vi "splash.vi"() -> ()   [LabVIEW 2010]
uses:
  <vilib>/Utility/miscctls.llb/LVRectTypeDef.ctl
  lib/Global 2.vi
  <vilib>/Platform/browser.llb/Open URL in Default Browser (string).vi
panel:
  out "msgs":cluster{"time stamp":timestamp, "t0":string}[](array[cluster]) {"time stamp" format="%<%.1X>T"}
  out "Bool3":bool
  out "Bool2":bool
  out "size(s)":i32 caption="шт"
  out "names":string[](array[string]) caption="Неотправленные"
  in  "Tab Control":T1(tab)
  out "Waveform Graph":waveform(i16)[](graph) caption="Последний кадр"
  out "Waveform Graph 2":waveform(i16)[](graph) caption="Последний кадр"
  out "XY Graph":cluster{dbl[], dbl[]}(graph) caption="неотправлено файлов"
  out "XY2":cluster{dbl[], dbl[]}(graph) caption="использование буфера"
  in  "indexhtm":bool
  out "Array":timestamp[](array[timestamp]) caption="Время событий" format="%<%.7X>T"
  out "Bool":bool
  in  "stop":bool
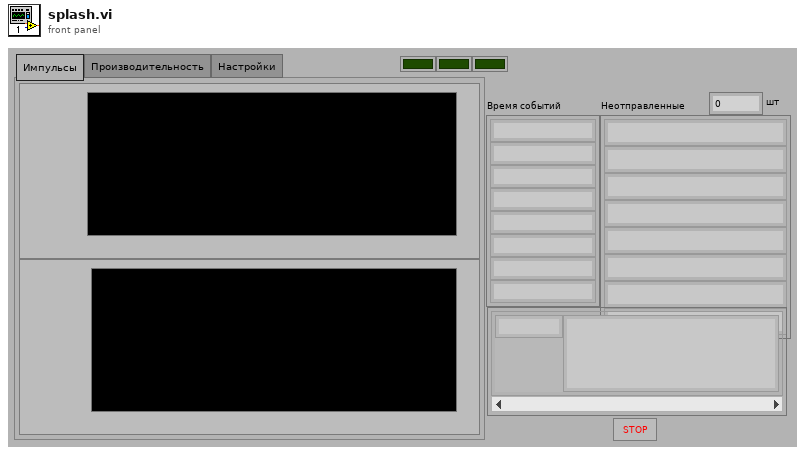
[diagram p1: front panel]
types:
  T1 = enum32{"Импульсы", "Производительность", "Настройки"}
  T2 = enum8{"Enabled", "Disabled", "Disabled and Grayed Out"}
  T3 = typedef "LVRectTypeDef.ctl" = cluster{"Left":i16, "Top":i16, "Right":i16, "Bottom":i16}
  T4 = cluster{"name":enum16{"sync", "phase_a", "phase_b", "phase_c", "ground"}, "num":i32}[]
  T5 = cluster{"seconds since 1Jan1904":timestamp, string}
  T6 = cluster{"seconds since 1Jan1904":timestamp, string}[]
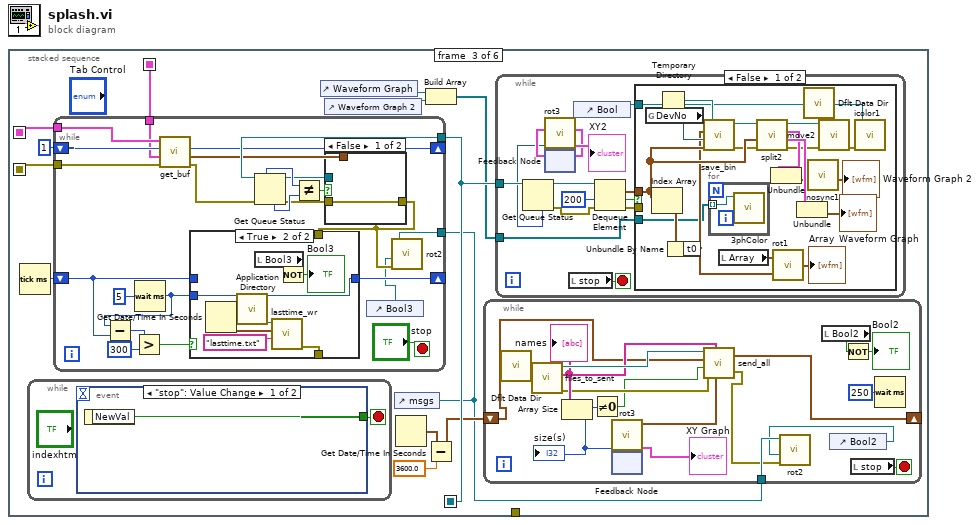
[diagram p0: block diagram]
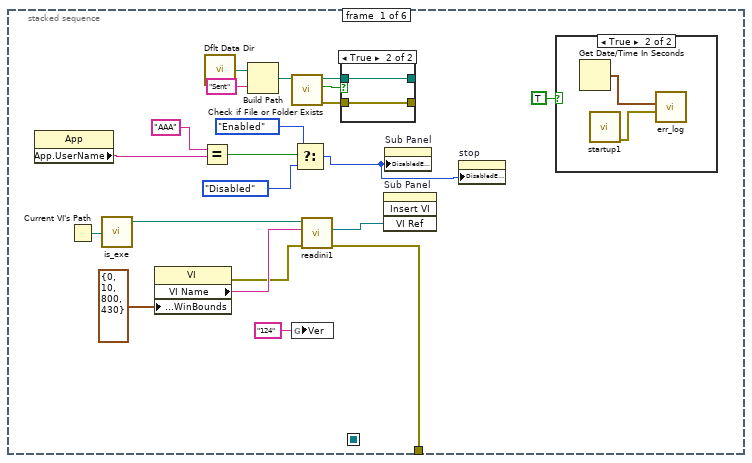
[diagram p2: hidden frame]
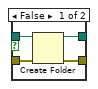
[diagram p4: hidden frame]
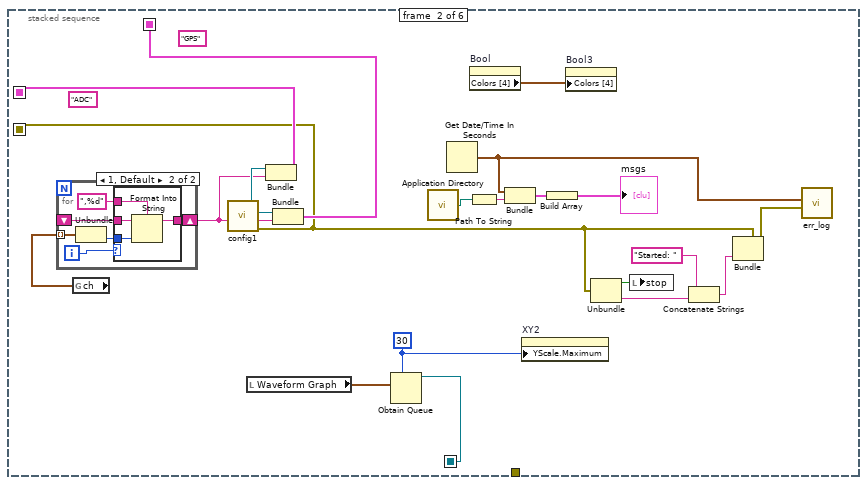
[diagram p5: hidden frame]
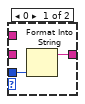
[diagram p6: hidden frame]
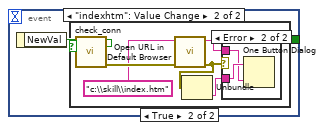
[diagram p7: hidden frame]
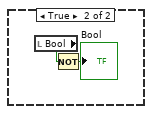
[diagram p10: hidden frame]
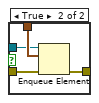
[diagram p12: hidden frame]
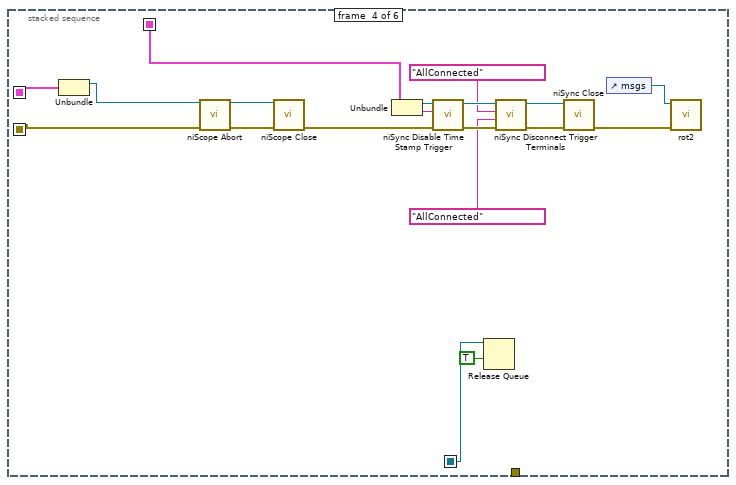
[diagram p13: hidden frame]
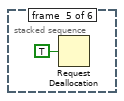
[diagram p14: hidden frame]
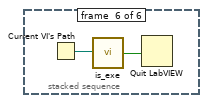
[diagram p15: hidden frame]
diagram:
  n1 = stacked-sequence {
    seq-local: [_ w35 _ _ _ _] -> [_ _ w76 w190 _ _]
    seq-local: [_ w51 _ _ _ _] -> [_ _ w75 w196 _ _]
    seq-local: [_ w45 _ _ _ _] -> [_ _ w73 w184 _ _]
    seq-local: [_ w46 _ _ _ _] -> [_ _ w72 w186 _ _]
    tunnel: [w18 _ _ _ _ _] -> _
    frame #0 {
      n2 = property class="App"() -> ("App.UserName"=w4:string)  [unwired: 2 in, 2 out]
      n3 = Current VI's Path() -> (path=w21:path)
      n4 = call "is_exe.vi"("path"=w21) -> ("ini path"=w19:path)  [unwired: 2 in, 2 out]
      n5 = property class="VI"("Front Panel.WinBounds"=T3 {"Left"=0, "Top"=10, "Right"=800, "Bottom"=430} ("Front Panel Window:Window Bounds")) -> (error out=w17:errorcluster, "VI Name"=w20:string)  [unwired: 2 in, 1 out]
      n6 = Equal?(x="ААА", y=w4) -> (x = y?=w7:bool)
      n7 = call <vilib>:"Dflt Data Dir.vi"() -> ("App:Default Data Directory"=w14:path)
      n8 = Build Path(base path=w14, name or relative path="Sent") -> (appended path=w12:path)
      n9 = call <vilib>:"Check if File or Folder Exists.vi"("path"=w12) -> ("error out"=w9:errorcluster, "file or folder exists?"=w11:bool, "dup path"=w10:path)  [unwired: 8 in]
      n10 = global write "Global 2.vi" "Ver"("124" ("Ver")) -> ()
      n11 = Select(t=T2."Enabled" ("Disabled"), s=w7, f=T2."Disabled" ("Disabled")) -> (s? t:f=w3:T2)
      n12 = call "readini1.vi"("error in (no error)"=w17, "section"=w20, "configuration file path"=w19) -> ("error out"=w18:errorcluster, "ini_reference out"=w15:refnum<vi>)  [unwired: 2 in, 1 out]
      n13 = case shown="True" w11 {
        tunnel: w10 -> [w27 w29]
        tunnel: w9 -> [w26 w28]
        tunnel: [w25 w29] -> _
        tunnel: [w24 w28] -> _
        frame False {
          n14 = Create Folder(path (use dialog)=w27, error in=w26) -> (created path=w25:path, error out=w24:errorcluster)  [unwired: 1 in, 1 out]
        }
        frame True {
        }
      }
      n15 = invoke on="Sub Panel" class="SubPanel" method="Insert VI"("VI Ref"=w15) -> ()  [unwired: 3 in, 4 out]
      n16 = property on="Sub Panel" class="SubPnl"("DisabledEnum"=w3) -> ()  [unwired: 2 in, 2 out]
      n17 = property on="stop" class="Bool (strict)"("DisabledEnum"=w3) -> ()  [unwired: 2 in, 2 out]
      n18 = case shown="True" TRUE {
        frame False {
        }
        frame True {
          n19 = Get Date/Time In Seconds() -> (seconds since 1Jan1904=w22:timestamp)
          n20 = call "startup1.vi"() -> ("error out"=w23:errorcluster)  [unwired: 7 in]
          n21 = call "err_log.vi"("error IO 2"=w23, "time stamp"=w22) -> ()  [unwired: 6 in]
        }
      }
    }
    frame #1 {
      (unwired) "GPS"
      w42 = 30 ("max queue size (-1, unlimited)")
      (unwired) "ADC"
      n22 = global read "Global 2.vi" "ch"() -> (w50:T4)
      n23 = for {
        shift-right: [w55] -> w43
        shift-left: _ -> [w54]
        tunnel: w50 -> [w57] mode=indexing
        i -> [w53]
        n24 = Unbundle(w57) -> ("num"=w56:i32)  [unwired: 1 out]
        n25 = case shown="1, Default" w53 {
          tunnel: w56 -> [w59 w63]
          tunnel: [w58 w62] -> w55
          tunnel: w54 -> [_ w61]
          tunnel: ",%d" -> [_ w60]
          frame 0 {
            n26 = Format Into String(w59) -> (resulting string=w58:string)  [unwired: 3 in, 1 out]
          }
          frame 1, Default {
            n27 = Format Into String(format string=w60, initial string=w61, w63) -> (resulting string=w62:string)  [unwired: 1 in, 1 out]
          }
        }
      }
      n28 = call "config1.vi"("ChList"=w43) -> ("error out"=w35:errorcluster, "trig"=w47:tag, "gps handle"=w48:refnum<k15>, "adc handle"=w49:refnum<k15>)  [unwired: 3 in]
      n29 = local read "Waveform Graph"() -> (w44:waveform(i16)[])
      n30 = Bundle("adc handle"=w49, w43) -> (w46:cluster{"adc handle":refnum<k15>, string})  [unwired: 1 in]
      n31 = Bundle("gps handle"=w48, "trig"=w47) -> (w45:cluster{"gps handle":refnum<k15>, "trig":tag})  [unwired: 1 in]
      n32 = Obtain Queue(max queue size (-1, unlimited)=w42, element data type=w44) -> (queue out=w51:refnum<queue>)  [unwired: 3 in, 2 out]
      n33 = call <vilib>:"Application Directory.vi"() -> ("Application Directory"=w39:path)
      n34 = Get Date/Time In Seconds() -> (seconds since 1Jan1904=w36:timestamp)
      n35 = Path To String(path=w39) -> (string=w41:string)
      n36 = property on="Bool" class="Bool (strict)"() -> ("Colors [4]"=w30:cluster{u32, u32}[])  [unwired: 2 in, 2 out]
      n37 = Bundle("seconds since 1Jan1904"=w36, w41) -> (w40:T5)  [unwired: 1 in]
      n38 = property on="XY2" class="XYGraph (strict)"("YScale.Maximum"=w42) -> ()  [unwired: 2 in, 2 out]
      n39 = Build Array(w40) -> (→"msgs":T6)
      n40 = property on="Bool3" class="Bool (strict)"("Colors [4]"=w30) -> ()  [unwired: 2 in, 2 out]
      n41 = Unbundle(w35) -> ("status"=w38:bool, "source"=w32:string)  [unwired: 1 out]
      n42 = local write "stop"(w38) -> ()
      n43 = Concatenate Strings("Started: " ("string"), w32) -> (w33:string)
      n44 = Bundle(cluster=w35, "source"=w33) -> (w34:errorcluster)  [unwired: 2 in]
      n45 = call "err_log.vi"("error IO 2"=w34, "time stamp"=w36) -> ()  [unwired: 6 in]
    }
    frame #2 {
      n46 = Tick Count (ms)() -> (millisecond timer value=w71:u32)
      n47 = while {
        stop <- w77 stop-if-true
        n48 = event shown="[0] \"stop\": Value Change" {
          selector: _ -> [_ _]
          dyn-events: _ -> [_ _]
          timeout: _ -> [_ _]
          tunnel: [w78 _] -> w77
          event "stop": Value Change {
            n49 = event-data() -> ("NewVal"=w78:bool)  [unwired: 1 in]
          }
          event "indexhtm": Value Change {
            n50 = event-data() -> ("NewVal"=w79:bool)  [unwired: 1 in]
            n51 = case shown="True" w79 {
              frame False {
              }
              frame True {
                n52 = call "check_conn.vi"() -> ("error out"=w81:errorcluster)  [unwired: 6 in, 1 out]
                n53 = call-poly <vilib>:"Open URL in Default Browser.vi"("error in (no error)"=w81, "URL"="c:\\skill\\index.htm") -> ("error out"=w84:errorcluster, "URL out"=w82:string)  [unwired: 4 in]
                n54 = Unbundle(w84) -> ("source"=w83:string)  [unwired: 2 out]
                n55 = case shown="Error" w84 {
                  tunnel: w83 -> [_ w86]
                  tunnel: w82 -> [_ w85]
                  frame No Error {
                  }
                  frame Error {
                    n56 = One Button Dialog(message=w86, button name ("OK")=w85) -> ()  [unwired: 1 out]
                  }
                }
              }
            }
          }
        }
      }
      n57 = control-ref of="Waveform Graph"() -> (w65:refnum<vi>)
      n58 = control-ref of="Waveform Graph 2"() -> (w66:refnum<vi>)
      n59 = control-ref of="msgs"() -> (w67:refnum<vi>)
      n60 = while {
        tunnel: w75 -> [w165]
        tunnel: w76 -> [w154]
        shift-right: [w158] -> _
        shift-left: 1 ("acquisition status out") -> [w157]
        tunnel: w73 -> [w145]
        tunnel: w72 -> [w146]
        shift-right: [w150] -> _
        shift-left: w71 -> [w149]
        tunnel: w67 -> [w144]
        stop <- "stop" stop-if-true
        n61 = Wait (ms)(milliseconds to wait=u32 5) -> (millisecond timer value=w148:u32)
        n62 = Subtract(x=w148, y=w149) -> (x-y=w153:u32)
        n63 = Greater?(x=w153, y=u32 300) -> (0:w152:bool)
        n64 = call "get_buf.vi"("error in"=w154, "Sync cluster"=w145, "acquisition status"=w157, "Scope Cluster"=w146) -> ("error out"=w155:errorcluster, "wfm"=w156:waveform(i16)[], "acquisition status out"=w158:i32)  [unwired: 1 in]
        n65 = Get Queue Status(queue=w165, error in (no error)=w155) -> (queue out=w161:refnum<queue>, max queue size=w164:i32, error out=w160:errorcluster, # elements in queue=w163:i32)  [unwired: 1 in, 4 out]
        n66 = Not Equal?(x=w164, y=w163) -> (x != y?=w162:bool)
        n67 = case shown="False" w162 {
          tunnel: w156 -> [_ w179]
          tunnel: w161 -> [_ w178]
          tunnel: w160 -> [w175 w177]
          tunnel: [w175 w176] -> w143
          frame False {
          }
          frame True {
            n68 = Enqueue Element(queue=w178, element=w179, error in (no error)=w177) -> (error out=w176:errorcluster)  [unwired: 1 in, 2 out]
          }
        }
        n69 = case shown="True" w152 {
          tunnel: [w167 w170] -> w150
          tunnel: w148 -> [_ w170]
          tunnel: w149 -> [w167 _]
          tunnel: [w166 w169] -> _
          tunnel: w143 -> [w166 _]
          frame False {
          }
          frame True {
            n70 = Get Date/Time In Seconds() -> (seconds since 1Jan1904=w173:timestamp)
            n71 = call <vilib>:"Application Directory.vi"() -> ("Application Directory"=w168:path)
            n72 = local read "Bool3"() -> (w172:bool)
            n73 = call "lasttime_wr.vi"("name or relative path"="lasttime.txt", "time stamp"=w173, "start Path"=w168) -> ("error out"=w169:errorcluster)  [unwired: 3 in, 1 out]
            n74 = Not(x=w172) -> (.not. x?=→"Bool3":bool)
          }
        }
        n75 = control-ref of="Bool3"() -> (w142:refnum<vi>)
        n76 = call "rot2.vi"("error in"=w143, "Bool Refnum"=w142, "Arr Refnum"=w144) -> ()  [unwired: 4 in, 1 out]
      }
      n77 = Get Date/Time In Seconds() -> (seconds since 1Jan1904=w70:timestamp)
      n78 = Build Array(w65, w66) -> (w64:refnum<vi>[])
      n79 = Subtract(x=w70, y=3600.0) -> (x-y=w69:timestamp)
      n80 = while {
        shift-right: [w92] -> _
        shift-left: w69 -> [w91]
        tunnel: w67 -> [w89]
        stop <- w105 stop-if-true
        n81 = call <vilib>:"Dflt Data Dir.vi"() -> ("App:Default Data Directory"=w103:path)
        n82 = call "files_to_sent.vi"("Directory"=w103) -> ("error IO"=w95:errorcluster, "names"=w96:string[], "directory dup"=w97:path)  [unwired: 4 in]
        "names" <- w96
        n83 = Array Size(array=w96) -> (size(s)=w94:i32)
        "size(s)" <- w94
        n84 = Not Equal To 0?(x=w94) -> (x != 0?=w93:bool)
        n85 = feedback #1() -> (w99:cluster{timestamp[], dbl[]})  [unwired: 1 in]
        n86 = call "rot3.vi"("y"=w94, "FB_In"=w99) -> ("XY_Graph"=→"XY Graph":cluster{dbl[], dbl[]}, "FB_Out"=w100:cluster{timestamp[], dbl[]}, "current time"=w90:timestamp)  [unwired: 3 in]
        n87 = feedback-in #1(w100) -> ()
        n88 = call "send_all.vi"("current time"=w90, "names"=w96, "error IO"=w95, "Boolean"=w93, "Time Stamp"=w91, "directory dup"=w97) -> ("error out"=w88:errorcluster, "last ses time"=w92:timestamp)
        n89 = local read "Bool2"() -> (w98:bool)
        n90 = control-ref of="Bool2"() -> (w87:refnum<vi>)
        n91 = call "rot2.vi"("error in"=w88, "Bool Refnum"=w87, "Arr Refnum"=w89) -> ()  [unwired: 4 in, 1 out]
        n92 = Not(x=w98) -> (.not. x?=→"Bool2":bool)
        n93 = local read "stop"() -> (w105:bool)
        n94 = Wait (ms)(milliseconds to wait=u32 250) -> ()  [unwired: 1 out]
      }
      n95 = while {
        tunnel: w75 -> [w116]
        tunnel: w64 -> [w106]
        stop <- w119 stop-if-true
        n96 = Get Queue Status(queue=w116) -> (queue out=w115:refnum<queue>, error out=w114:errorcluster, # elements in queue=w108:i32)  [unwired: 2 in, 5 out]
        n97 = feedback #2() -> (w110:cluster{timestamp[], dbl[]})  [unwired: 1 in]
        n98 = call "rot3.vi"("y"=w108, "FB_In"=w110) -> ("XY_Graph"=→"XY2":cluster{dbl[], dbl[]}, "FB_Out"=w109:cluster{timestamp[], dbl[]})  [unwired: 3 in, 1 out]
        n99 = feedback-in #2(w109) -> ()
        n100 = local read "stop"() -> (w119:bool)
        n101 = control-ref of="Bool"() -> (w107:refnum<vi>)
        n102 = Dequeue Element(queue=w115, timeout in ms (-1)=200, error in (no error)=w114) -> (element=w113:waveform(i16)[], timed out?=w117:bool, error out=w112:errorcluster)  [unwired: 1 out]
        n103 = case shown="False" w117 {
          tunnel: w113 -> [w136 _]
          tunnel: w112 -> [_ _]
          tunnel: w107 -> [w121 _]
          tunnel: w106 -> [w120 _]
          frame False {
            n104 = global read "Global 2.vi" "DevNo"() -> (w130:i32)
            n105 = Index Array(array=w136) -> (element=w135:waveform(i16))  [unwired: 1 in]
            n106 = Temporary Directory() -> (w128:path)
            n107 = Unbundle By Name(w135) -> ("t0"=w129:timestamp)
            n108 = call "save_bin.vi"("SigArray"=w136, "DevNo"=w130, "timestamp"=w129, "start path"=w128) -> ("error out"=w125:errorcluster, "final Path"=w126:path)  [unwired: 2 in]
            n109 = for {
              tunnel: w120 -> [w139] mode=indexing
              n110 = call "3phColor.vi"("Waveform Graph 2"=w139) -> ()  [unwired: 7 in]
            }
            n111 = local read "Array"() -> (w133:timestamp[])
            n112 = call "split2.vi"("error in"=w125, "Waveforms"=w136, "full file path"=w126) -> ("error out"=w124:errorcluster, "compressed"=w138:cluster{"appended path":path, waveform(i16)[]}, "first"=w137:cluster{"appended path":path, waveform(i16)[]})  [unwired: 2 in]
            n113 = Unbundle(w137) -> (w131:waveform(i16)[])  [unwired: 1 out]
            n114 = call "rot1.vi"("t0"=w129, "Array"=w133) -> ("Array 2"=→"Array":timestamp[])
            n115 = Unbundle(w138) -> (→"Waveform Graph":waveform(i16)[])  [unwired: 1 out]
            n116 = call <vilib>:"Dflt Data Dir.vi"() -> ("App:Default Data Directory"=w127:path)
            n117 = call "nosync1.vi"("h 2"=w131) -> ("h 3"=→"Waveform Graph 2":waveform(i16)[])  [unwired: 6 in]
            n118 = call "move2.vi"("error in (no error)"=w124, "dst dir"=w127, "full file path"=w126) -> ("error out"=w122:errorcluster)  [unwired: 4 in]
            n119 = call "icolor1.vi"("error in (no error)"=w122, "Bool Refnum"=w121) -> ()  [unwired: 6 in]
          }
          frame True {
            n120 = local read "Bool"() -> (w140:bool)
            n121 = Not(x=w140) -> (.not. x?=→"Bool":bool)
          }
        }
      }
    }
    frame #3 {
      n122 = Unbundle(w186) -> ("adc handle"=w185:refnum<k15>)  [unwired: 1 out]
      n123 = call <instrlib>:"niScope Abort.vi"("instrument handle"=w185, "error in"=w190) -> ("instrument handle out"=w198:refnum<k15>, "error out"=w197:errorcluster)  [unwired: 12 in]
      n124 = call <instrlib>:"niScope Close.vi"("instrument handle"=w198, "error in"=w197) -> ("error out"=w191:errorcluster)  [unwired: 13 in]
      n125 = Unbundle(w184) -> ("gps handle"=w183:refnum<k15>, "trig"=w182:tag)
      n126 = call <instrlib>:"niSync Disable Time Stamp Trigger.vi"("error in (no error)"=w191, "terminal"=w182, "instrument handle"=w183) -> ("error out"=w194:errorcluster, "instrument handle out"=w195:refnum<k15>)  [unwired: 6 in]
      n127 = Release Queue(queue=w196, force destroy? (F)=TRUE) -> ()  [unwired: 1 in, 3 out]
      n128 = call <instrlib>:"niSync Disconnect Trigger Terminals.vi"("error in (no error)"=w194, "destination terminal"="AllConnected", "source terminal"="AllConnected", "instrument handle"=w195) -> ("error out"=w193:errorcluster, "instrument handle out"=w192:refnum<k15>)  [unwired: 6 in]
      n129 = call <instrlib>:"niSync Close.vi"("error in (no error)"=w193, "instrument handle"=w192) -> ("error out"=w181:errorcluster)  [unwired: 9 in]
      n130 = control-ref of="msgs"() -> (w180:refnum<vi>)
      n131 = call "rot2.vi"("error in"=w181, "Arr Refnum"=w180) -> ()  [unwired: 5 in, 1 out]
    }
    frame #4 {
      n132 = Request Deallocation(TRUE ("flag")) -> ()
    }
    frame #5 {
      n133 = Current VI's Path() -> (path=w201:path)
      n134 = call "is_exe.vi"("path"=w201) -> ("exe?"=w200:bool)  [unwired: 2 in, 2 out]
      n135 = Quit LabVIEW(quit? (T)=w200) -> ()
    }
  }
